vi "Format Digital Control.vi"(6 "Format String":string, 8 "error in":errorcluster, 11 "GObject in":refnum<vi>) -> (0 "error out":errorcluster, 2 "Successful":bool)   [LabVIEW 2019, in "Quick Format QD.lvlib"]
doc: "Formats a digital control based on the given Format String."
uses:
  Quick Format QD.lvlib
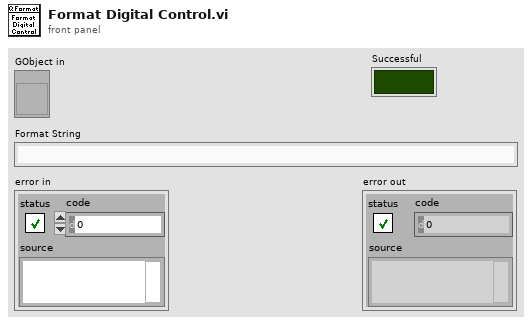
[diagram p1: front panel]
types:
  T1 = typedef "LVNumericRepresentation.ctl" = enum32{"Extended Precision", "Double Precision", "Single Precision", "Long", "Word", "Byte", "Unsigned Long", "Unsigned Word", "Unsigned Byte", "Complex Extended", "Complex Double", "Complex Single", "Quad", "Unsigned Quad", "Fixed-Point"}
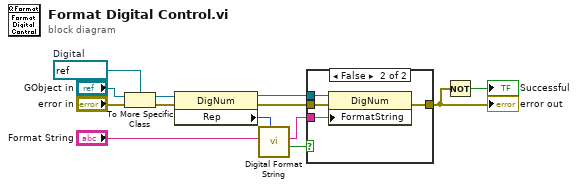
[diagram p0: block diagram]
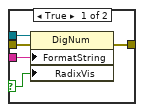
[diagram p2: hidden frame]
diagram:
  w9 = refnum<vi> refnum  # Digital
  n1 = To More Specific Class(target class=w9, reference="GObject in", error in="error in") -> (specific class reference=w8:refnum<vi>, error out=w13:errorcluster)
  n2 = property on="Property Node" class="DigNum"(reference=w8, error in=w13) -> (reference out=w2:refnum<vi>, error out=w10:errorcluster, "Rep"=w5:T1)
  n3 = call "Digital Format String.vi"("Representation"=w5, "Format String in"="Format String") -> ("Force Radix Visible"=w1:bool, "Format String out"=w3:string)  [unwired: 8 in]
  n4 = case shown="False" w1 {
    selector: w1 -> [w14 _]
    tunnel: [w18 w22] -> w11
    tunnel: w3 -> [w16 w20]
    tunnel: w2 -> [w15 w19]
    tunnel: w10 -> [w17 w21]
    frame True {
      n5 = property on="Property Node" class="DigNum"(reference=w15, error in=w17, "FormatString"=w16, "RadixVis"=w14) -> (error out=w18:errorcluster)  [unwired: 1 out]
    }
    frame False {
      n6 = property on="Property Node" class="DigNum"(reference=w19, error in=w21, "FormatString"=w20) -> (error out=w22:errorcluster)  [unwired: 1 out]
    }
  }
  "error out" <- w11
  n7 = Not(x=w11) -> (.not. x?=→"Successful":bool)
